vi "MC5e Remove Squad from Unit.vi"(7 "index of squad to reduce":i32, 8 "error in":errorcluster, 9 "# to remove":u16, 11 "Unit Index":i32) -> (0 "error out":errorcluster)   [LabVIEW 2020]
uses:
  MC5e Unit_Manager_Modes.ctl
  MC5e Editor modes.ctl
  MC5e Squad_Manager_Modes.ctl
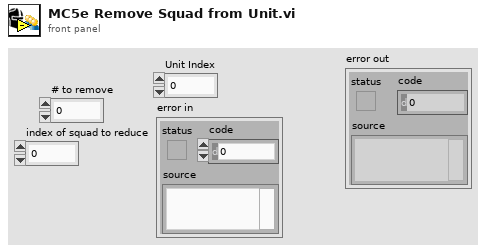
[diagram p1: front panel]
types:
  T1 = typedef "MC5e Unit.ctl" = cluster{"Unit Fatigue Level":enum16{"Not Fatigued", "Fatigued", "Seriously Fatigued"}, "Flying Unit":bool, "Mounted Unit":bool, "Defending from Stronghold":bool, "Difficult Terrain Types":T2, "Squads in Unit":T3[], "Unit Info":T5, "Range":i32, "BR":i32, "Speed":i32, "Morale":i32, "Current BR":i32, "Location":T6, "Capacity %":i32}
  T2 = typedef "MC5e Terrain types.ctl" = i32[]
  T3 = typedef "MC5e Squad_Info.ctl" = cluster{"Squad Name":string, "# Soldiers":u16, "Battle Rating":u16, "Flying":bool, "Mounted":bool, "Speed":u16, "Range":u16, "Morale":i32, "Max Endurance":u16, "Current Endurance":i32, "Size":T4, "Space Taken":u16, "Difficult Terrain":i32[], "CR":u16, "Special / Notes":string}
  T4 = typedef "MC5e Size_Categories.ctl" = enum16{"Tiny", "Small", "Medium", "Large", "Huge", "Gargantuan"}
  T5 = typedef "MC5e Unit Header.ctl" = cluster{"Unit Name":string, "Unit Commander":string, "Morale Mod":i32, "BR Mod":i32, "Defense Mod":i32, "Speed Mod":i32, "Unit Notes":string, "Attack Mod":i32, "Unit Wins+ Losses-":i32, "Commander Charisma Bonus":i32}
  T6 = typedef "Location.ctl" = cluster{"X coordinate":dbl, "Y coordinate":dbl}
  T7 = typedef "MC5e Editor modes.ctl" = enum16{"Add New", "Copy Selected", "Delete Selected", "Edit Selected"}
  T8 = typedef "MC5e Unit_Manager_Modes.ctl" = enum16{"Initialize", "Add Unit", "Delete Unit", "Get Unit", "Load Set", "Replace Unit"}
  T9 = typedef "MC5e Squad_Manager_Modes.ctl" = enum16{"Initialize", "Add Squad", "Delete Squad", "Get Squad", "Replace Squad", "Load Set"}
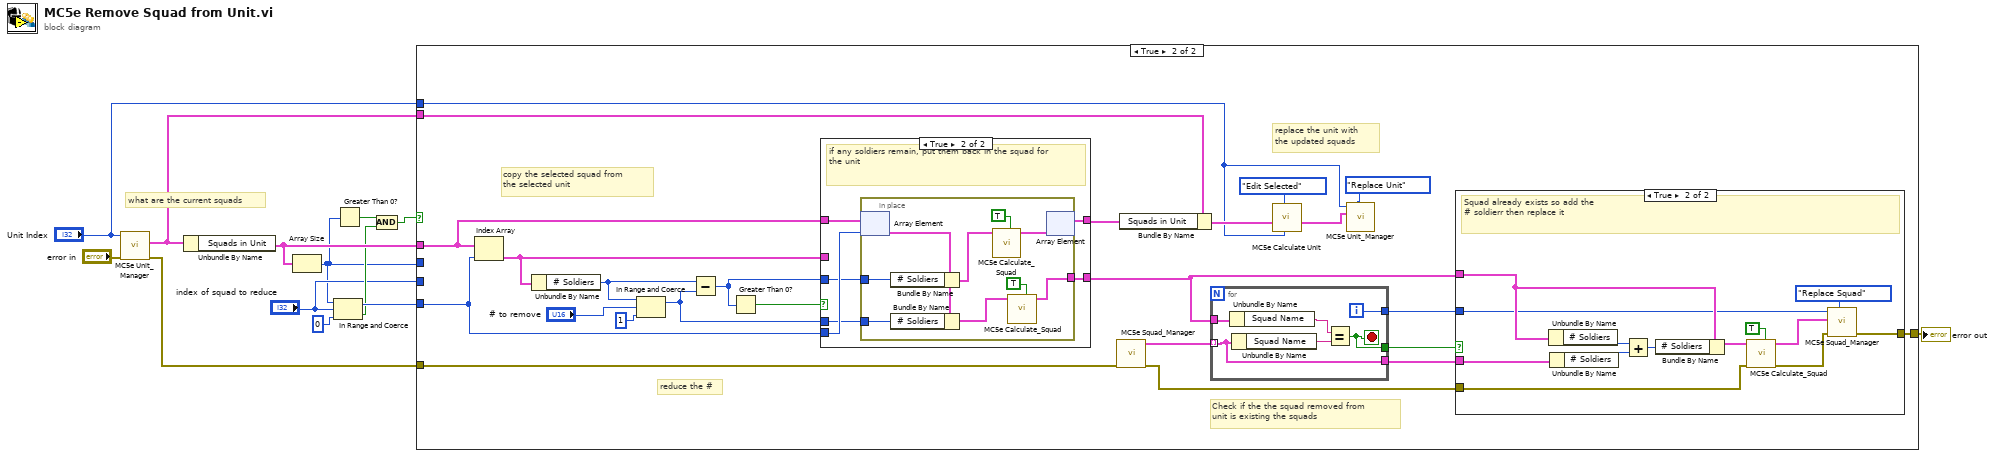
[diagram p0: block diagram]
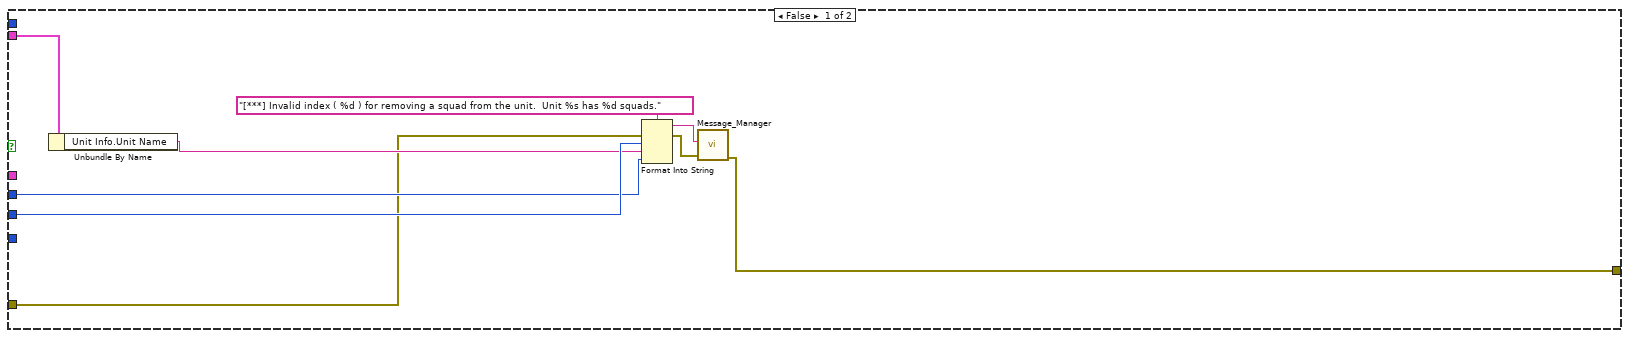
[diagram p2: hidden frame]
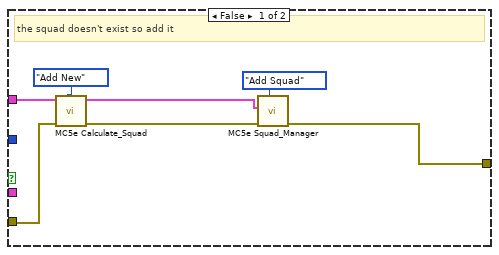
[diagram p3: hidden frame]
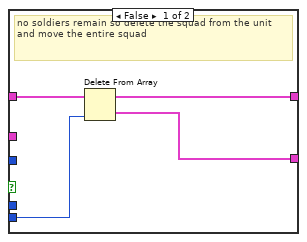
[diagram p4: hidden frame]
diagram:
  # "what are the current squads"
  n1 = call "MC5e Unit_Manager.vi"("error in"="error in", "index (get/delete/replace)"="Unit Index") -> ("error out"=w9:errorcluster, "Unit"=w13:T1)  [unwired: 6 in, 2 out]
  n2 = Unbundle By Name(w13) -> ("Squads in Unit"=w8:T3[])
  n3 = Array Size(array=w8) -> (size(s)=w1:i32)
  n4 = In Range and Coerce(upper limit=w1, x="index of squad to reduce", lower limit=0) -> (coerced(x)=w5:i32, In Range?=w3:bool)
  n5 = Greater Than 0?(x=w1) -> (x > 0?=w7:bool)
  n6 = And(x=w7, y=w3) -> (x .and. y?=w4:bool)
  n7 = case shown="True" w4 {
    tunnel: w13 -> [w18 w39]
    tunnel: "Unit Index" -> [_ w34]
    tunnel: [w14 w33] -> w10
    tunnel: w9 -> [w15 w31]
    tunnel: w8 -> [_ w24]
    tunnel: w5 -> [_ w23]
    tunnel: "index of squad to reduce" -> [w19 _]
    tunnel: w1 -> [w17 _]
    frame False {
      n8 = Unbundle By Name(w18) -> ("Unit Info.Unit Name"=w16:string)
      n9 = Format Into String(format string="[***] Invalid index ( %d ) for removing a squad from the unit.  Unit %s has %d squads.", error in=w15, w19, w16, w17) -> (resulting string=w21:string, error out=w20:errorcluster)  [unwired: 1 in]
      n10 = call "Message_Manager.vi"("error in"=w20, "New Entry"=w21) -> ("error out"=w14:errorcluster)  [unwired: 5 in, 4 out]
    }
    frame True {
      # "Check if the the squad removed from \nunit is existing the squads"
      # "replace the unit with \nthe updated squads"
      # "reduce the #"
      # "copy the selected squad from \nthe selected unit"
      n11 = Index Array(array=w24, index=w23) -> (element=w25:T3)
      n12 = Unbundle By Name(w25) -> ("# Soldiers"=w44:u16)
      n13 = In Range and Coerce(upper limit=w44, x="# to remove", lower limit=u16 1) -> (coerced(x)=w30:u16)  [unwired: 1 out]
      n14 = Subtract(x=w44, y=w30) -> (x-y=w42:u16)
      n15 = Greater Than 0?(x=w42) -> (x > 0?=w43:bool)
      n16 = case shown="True" w43 {
        tunnel: w42 -> [_ w81]
        tunnel: w23 -> [w75 w82]
        tunnel: [w73 w77] -> w40
        tunnel: [w74 w80] -> w29
        tunnel: w25 -> [_ _]
        tunnel: w30 -> [_ w79]
        tunnel: w24 -> [w76 w78]
        frame False {
          # "no soldiers remain so delete the squad from the unit and move the entire squad"
          n17 = Delete From Array(array=w76, index=w75) -> (deleted portion=w74:T3, array with subset deleted=w73:T3[])  [unwired: 1 in]
        }
        frame True {
          # "if any soldiers remain, put them back in the squad for the unit"
          n18 = in-place {
            in-place-border: w81 -> [w91]
            in-place-border: [w87] -> w80
            in-place-border: w79 -> [w90]
            n19 = in-place-array #1(w78, w82) -> (w84:T3)
            n20 = Bundle By Name(cluster=w84, "# Soldiers"=w91) -> (w86:T3)
            n21 = Bundle By Name(cluster=w84, "# Soldiers"=w90) -> (w83:T3)
            n22 = call "MC5e Calculate_Squad.vi"("Skip Name Check (F)"=TRUE, "Input Squad"=w86) -> ("output squad"=w85:T3)  [unwired: 7 in, 2 out]
            n23 = call "MC5e Calculate_Squad.vi"("Skip Name Check (F)"=TRUE, "Input Squad"=w83) -> ("output squad"=w87:T3)  [unwired: 7 in, 2 out]
            n24 = in-place-array #1(w85) -> (w77:T3[])  [unwired: 1 out]
          }
        }
      }
      n25 = call "MC5e Squad_Manager.vi"("error in"=w31) -> ("error out"=w32:errorcluster, "All Squads Out"=w38:T3[])  [unwired: 7 in, 2 out]
      n26 = Bundle By Name(cluster=w39, "Squads in Unit"=w40) -> (w36:T1)
      n27 = for {
        tunnel: w38 -> [w67] mode=indexing
        tunnel: w29 -> [w72]
        tunnel: [w69] -> w28
        tunnel: [w68] -> w27
        tunnel: [w67] -> w26
        i -> [w68]
        stop <- w69 stop-if-true
        n28 = Unbundle By Name(w72) -> ("Squad Name"=w70:string)
        n29 = Unbundle By Name(w67) -> ("Squad Name"=w71:string)
        n30 = Equal?(x=w70, y=w71) -> (x = y?=w69:bool)
      }
      n31 = call "MC5e Calculate Unit.vi"("index"=w34, "Mode"=MC5e_Editor_modes."Edit Selected", "Unit In"=w36) -> ("Unit Out"=w35:T1)  [unwired: 5 in, 3 out]
      n32 = call "MC5e Unit_Manager.vi"("Mode (Get)"=MC5e_Unit_Manager_Modes."Replace Unit", "Unit In (Add/Replace)"=w35, "index (get/delete/replace)"=w34) -> ()  [unwired: 5 in, 4 out]
      n33 = case shown="True" w28 {
        tunnel: w29 -> [w48 w66]
        tunnel: w27 -> [_ w65]
        tunnel: [w49 w63] -> w33
        tunnel: w32 -> [w51 w55]
        tunnel: w26 -> [_ w59]
        frame False {
          # "the squad doesn't exist so add it"
          n34 = call "MC5e Calculate_Squad.vi"("Mode"=MC5e_Editor_modes."Add New", "error in"=w51, "Input Squad"=w48) -> ("error out"=w50:errorcluster, "output squad"=w47:T3)  [unwired: 6 in, 1 out]
          n35 = call "MC5e Squad_Manager.vi"("Mode (Get)"=MC5e_Squad_Manager_Modes."Add Squad", "error in"=w50, "Squad in (add/replace)"=w47) -> ("error out"=w49:errorcluster)  [unwired: 5 in, 3 out]
        }
        frame True {
          # "Squad already exists so add the\n# soldierr then replace it"
          n36 = Unbundle By Name(w66) -> ("# Soldiers"=w61:u16)
          n37 = Unbundle By Name(w59) -> ("# Soldiers"=w62:u16)
          n38 = Add(x=w61, y=w62) -> (x+y=w60:u16)
          n39 = Bundle By Name(cluster=w66, "# Soldiers"=w60) -> (w57:T3)
          n40 = call "MC5e Calculate_Squad.vi"("Skip Name Check (F)"=TRUE, "error in"=w55, "Input Squad"=w57) -> ("error out"=w54:errorcluster, "output squad"=w56:T3)  [unwired: 6 in, 1 out]
          n41 = call "MC5e Squad_Manager.vi"("Mode (Get)"=MC5e_Squad_Manager_Modes."Replace Squad", "error in"=w54, "Squad in (add/replace)"=w56, "index (get/delete/replace)"=w65) -> ("error out"=w63:errorcluster)  [unwired: 4 in, 3 out]
        }
      }
    }
  }
  "error out" <- w10
